vi "Write Remaining Length (bytes).vi"(10 "Remaining Length (bytes)":u32, 11 "ControlPacket in":refnum<class "ControlPacket.lvclass">) -> (3 "ControlPacket out":refnum<class "ControlPacket.lvclass">)   [LabVIEW 2013, in "MQTT_Control_Packets.lvlib" / "ControlPacket.lvclass"]
uses:
  ControlPacket.lvclass
  ControlPacket.lvclass/ControlPacket.ctl
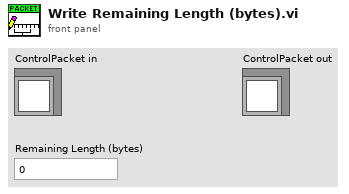
[diagram p1: front panel]
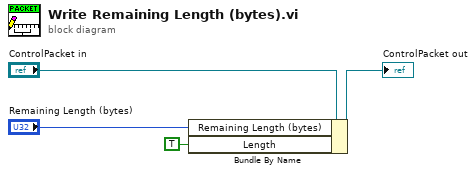
[diagram p0: block diagram]
diagram:
  n1 = Bundle By Name(cluster="ControlPacket in", "Remaining Length (bytes)"="Remaining Length (bytes)", "Length"=TRUE) -> (→"ControlPacket out":refnum<class "ControlPacket.lvclass">)
